vi "InitMatlabEventStream.vi"(8 "error in":errorcluster, 11 "ExpID":string) -> (0 "error out":errorcluster)   [LabVIEW 2017]
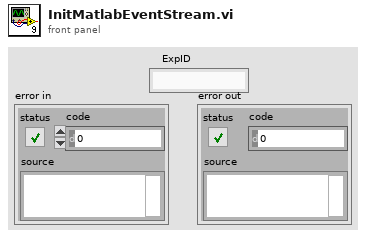
[diagram p1: front panel]
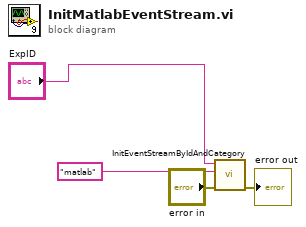
[diagram p0: block diagram]
diagram:
  n1 = call "InitEventStreamByIdAndCategory.vi"("error in"="error in", "Category"="matlab", "ID"="ExpID") -> ("error out"=→"error out":errorcluster)  [unwired: 7 in, 1 out]
